vi "VXM Main Test App.vi"() -> ()   [LabVIEW 2017]
doc: "Simple Qued Message Handler type of state machine.\nAlways use this template if the VI is a UI used by a user and it is more complex than a dialog.\n(Unless you're usig something more advanced like Actor Framework)\n\nBolder Software LLC"
uses:
  Classes/UI ExecutionCtrls/UI ExecutionCtrls.lvclass
  Classes/UI MotionStatus/UI MotionStatus.lvclass
  Support/MessageAPI/MoveAllAbsolute.ctl
  Classes/UI ExecutionCtrls/MotionExecutionCtrlRefs.ctl
  Classes/UI MotionStatus/MotionStatusLEDCtrlRefs.ctl
  Classes/UI MotionStatus/PositonIndicatorsCtrlRefs.ctl
  Support/MessageQue/MessageQue.lvlib
  Support/UserEvent-ExitEventLoop/UserEvent-ExitEventLoop.lvlib
panel:
  out "Home Established":bool
  in  "Polarization":u16(ring) items=["Vertical", "Horizontal"]
  in  "Move to Pos.":bool
  in  "Position":i32=1 caption="Antenna\nPosition" min=0 max=15 step=1
  in  "clear":bool
  out "UI Messages":string
  in  "MoveAllAbsolute":bool
  out "testing 2":bool
  in  "Stop Motion":bool
  out "T moving":bool
  out "Z moving":bool
  out "Y moving":bool
  out "X moving":bool
  out "Position,steps 4":sgl caption="Angle, degrees"
  out "Position,steps 3":sgl caption="Z Position, mm"
  out "Position,steps":sgl caption="Y Position, mm"
  out "Position,steps":sgl caption="X Position, mm"
  in  "T Jog, steps":i32 caption="T Jog distance, steps"
  in  "Z Jog, steps":i32 caption="Z Jog distance, steps"
  in  "Y Jog, steps":i32 caption="Y Jog distance, steps"
  in  "X Jog, steps":i32 caption="X Jog distance, steps"
  in  "FindHomeAll":bool
  in  "HomeAll":bool
  in  "T Home Button":bool
  in  "T Jog Neg.":bool
  in  "T Jog Pos.":bool
  in  "Set T Position, Deg.":dbl format="%.4f"
  in  "Z Home Button":bool
  in  "Z Jog Neg.":bool
  in  "Z Jog Pos.":bool
  in  "Set Z Position, mm":dbl format="%.4f"
  in  "Y Home Button":bool
  in  "Y Jog Neg.":bool
  in  "Y Jog Pos.":bool
  in  "Set Y Position, mm":dbl format="%.4f"
  in  "X Home Button":bool
  in  "X Jog Neg.":bool
  in  "X Jog Pos.":bool
  in  "Set X Position, mm":dbl format="%.4f"
  in  "Generate \"DAQ\" Loop TestError":bool
  in  "test error":errorcluster
  in  "Generate \"Main\" Loop TestError":bool
  out "i event":i32=6 caption="ievent"
  out "Command":string
  out "i main":i32=6
  # "Could put jog size control\non FP here to easily \nadjust jog and implement\nrelative moves trough the\njog buttons."
  # "Could set ini file as\nmotion / no motion\nand certain controls\nwould change context"
  # "combine this with Antenna Test"
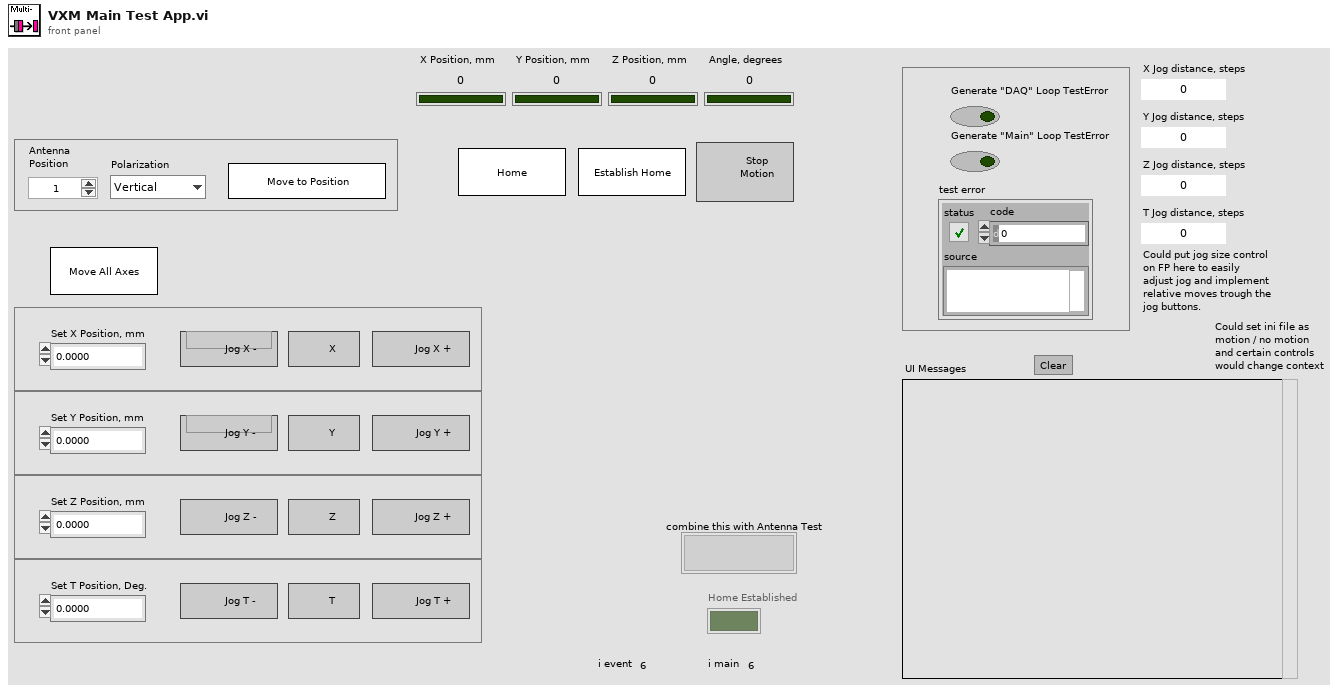
[diagram p1: front panel]
types:
  T1 = cluster{"ExecCtrls":refnum<class "UI ExecutionCtrls.lvclass">, "StatusInds":refnum<class "UI MotionStatus.lvclass">}
  T2 = typedef "MultipleMessageQues vxm.ctl" = cluster{"Main que":T3, "Error que":T3, "VXM Svc que":T3, "Listener que":T3, "VXM ACK que":T3, "DAQ que":T3}
  T3 = typedef "MessageQue.lvlib/MessageQue.ctl" = refnum<queue>
  T4 = typedef "MoveAllAbsolute.ctl" = cluster{"MoveType":string, "Move Params":dbl[]}
  T5 = typedef "PositonIndicatorsCtrlRefs.ctl" = cluster{"XPosition,steps":refnum<vi>, "YPosition,steps":refnum<vi>, "ZPosition,steps":refnum<vi>, "TPosition,steps":refnum<vi>}
  T6 = typedef "MotionStatusLEDCtrlRefs.ctl" = cluster{"Y moving":refnum<vi>, "Z moving":refnum<vi>, "T moving":refnum<vi>, "X moving":refnum<vi>}
  T7 = typedef "MotionExecutionCtrlRefs.ctl" = cluster{"MoveAllAbsolute":refnum<vi>, "Move to Pos.":refnum<vi>, "HomeAll":refnum<vi>, "FindHomeAll":refnum<vi>, "X Jog Pos.":refnum<vi>, "X Jog Neg.":refnum<vi>, "Y Jog Pos.":refnum<vi>, "Y Jog Neg. ":refnum<vi>, "Z Jog Pos.":refnum<vi>, "Z Jog Neg.":refnum<vi>, "T Jog Pos.":refnum<vi>, "T Jog Neg.":refnum<vi>, "X Home Button":refnum<vi>, "Y Home Button":refnum<vi>, "Z Home Button":refnum<vi>, "T Home Button":refnum<vi>}
  T8 = typedef "UIMessage.ctl" = cluster{"EventCode":i32, "Numeric":dbl, "String":string, "Variant":variant}
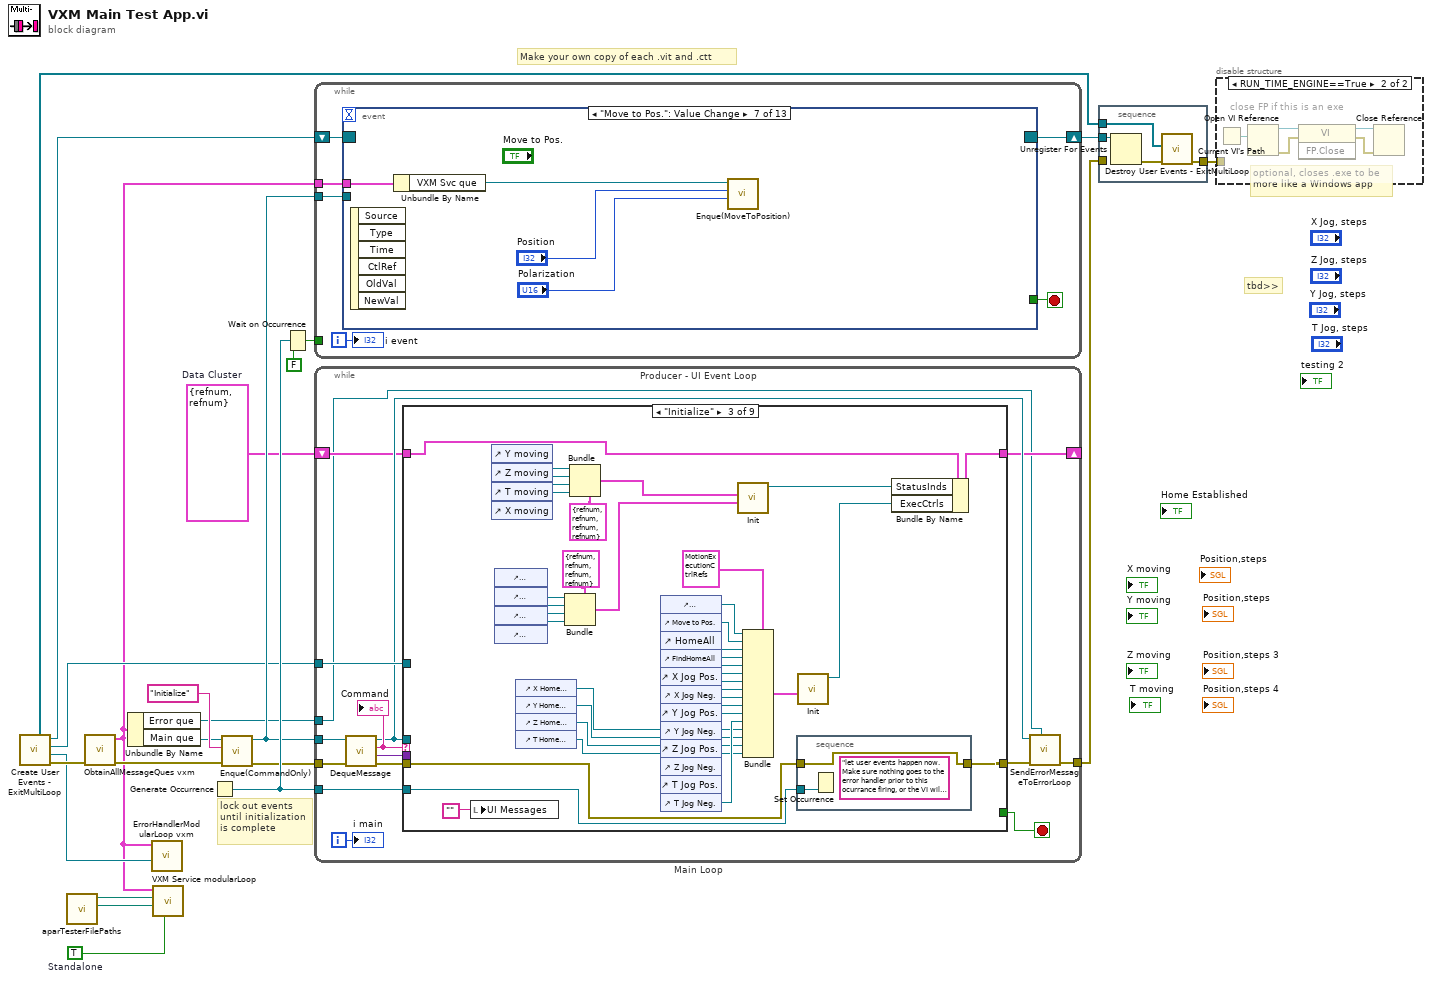
[diagram p0: block diagram]
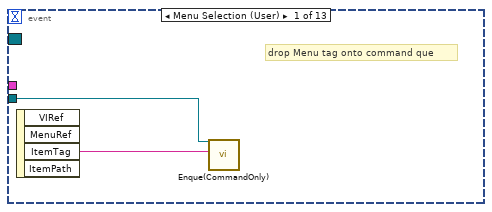
[diagram p3: hidden frame]
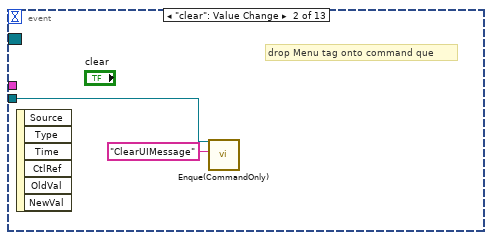
[diagram p4: hidden frame]
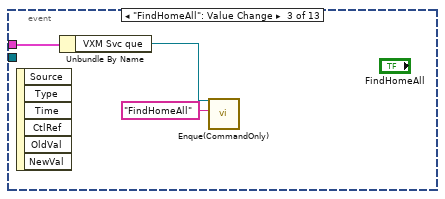
[diagram p5: hidden frame]
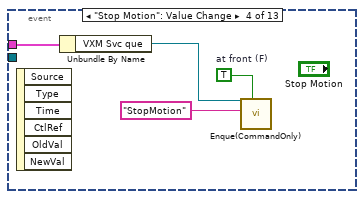
[diagram p6: hidden frame]
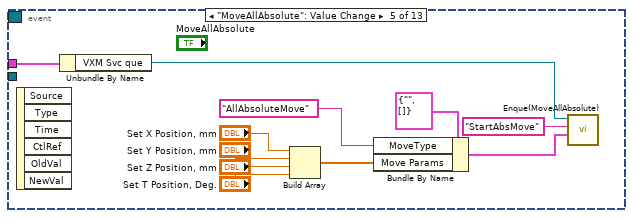
[diagram p7: hidden frame]
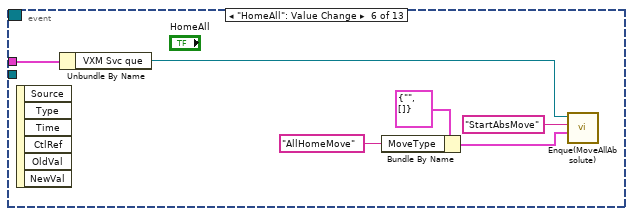
[diagram p8: hidden frame]
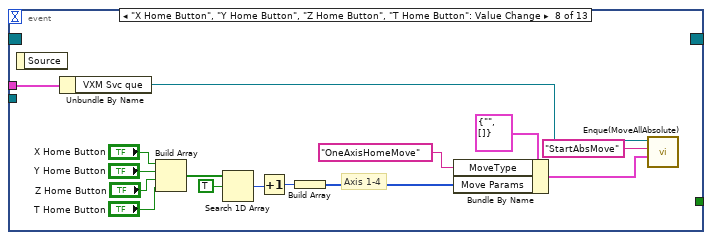
[diagram p9: hidden frame]
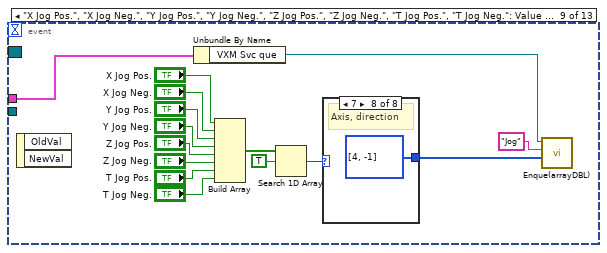
[diagram p10: hidden frame]
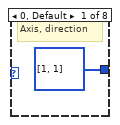
[diagram p11: hidden frame]
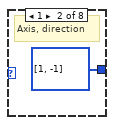
[diagram p12: hidden frame]
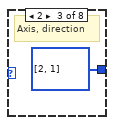
[diagram p13: hidden frame]
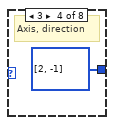
[diagram p14: hidden frame]
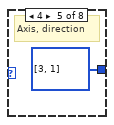
[diagram p15: hidden frame]
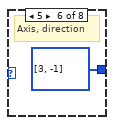
[diagram p16: hidden frame]
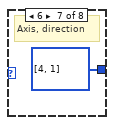
[diagram p17: hidden frame]
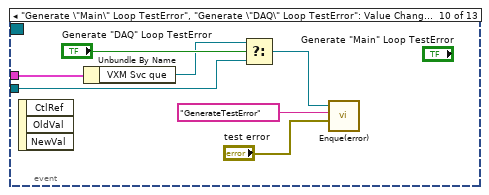
[diagram p18: hidden frame]
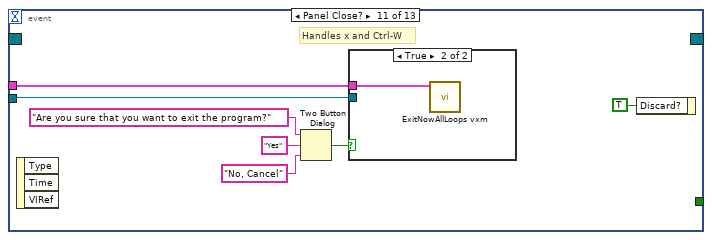
[diagram p19: hidden frame]
diagram:
  w1 = TRUE  # Standalone
  w13 = T1 {"ExecCtrls"=refnum, "StatusInds"=refnum}  # Data Cluster
  # "tbd>>"
  # "Make your own copy of each .vit and .ctt"
  # "lock out events\nuntil initialization\nis complete"
  # "optional, closes .exe to be \nmore like a Windows app"
  n1 = call "Create User Events - ExitMultiLoop.vi"() -> ("error out"=w12:errorcluster, "ExitALLLoops event out"=w5:refnum<user-event>, "ExitEventLoop event out"=w6:refnum<user-event>, "Events Registration Refnum"=w16:refnum<event-registration>, "user event array"=w7:refnum<user-event>[])  [unwired: 7 in]
  n2 = call "aparTesterFilePaths.vi"() -> ("Config File Path Motion"=w3:path, "Config File Path"=w2:path)  [unwired: 6 in, 4 out]
  n3 = call "ObtainAllMessageQues vxm.vi"("error in"=w12) -> ("error out"=w11:errorcluster, "MessageQues"=w4:T2)  [unwired: 9 in]
  n4 = Unbundle By Name(w4) -> ("Error que"=w8:T3, "Main que"=w10:T3)
  n5 = call "ErrorHandlerModularLoop vxm.vi"("exit event source"=w5, "MessageQues"=w4) -> ()  [unwired: 9 in, 1 out]
  n6 = call "VXM Service modularLoop.vi"("Standalone"=w1, "Motion Cfg File path"=w3, "Cfg File path"=w2, "MessageQues"=w4) -> ()  [unwired: 8 in]
  n7 = Generate Occurrence() -> (w22:refnum<k4>)
  n8 = call "Enque(CommandOnly).vi"("error in"=w11, "Message Command"="Initialize", "Message que"=w10) -> ("error out"=w18:errorcluster, "Message que out"=w17:T3)  [unwired: 7 in]
  n9 = Wait on Occurrence(1:FALSE ("ignore previous (T)"), 2:w22) -> (0:w15:bool)  [unwired: 1 in]
  n10 = while "Producer - UI Event Loop" {
    shift-right: [w24] -> w21
    shift-left: w16 -> [w25]
    tunnel: w17 -> [w27]
    tunnel: w15 -> [_]
    tunnel: w4 -> [w23]
    i -> [w28]
    stop <- w26 stop-if-true
    n11 = event shown="[6] \"Move to Pos.\": Value Change" {
      selector: w25 -> [_ _ _ _ _ _ _ _ _ _ _ _ _]
      dyn-events: [_ _ _ _ _ _ _ _ _ _ _ _ _] -> w24
      timeout: _ -> [_ _ _ _ _ _ _ _ _ _ _ _ _]
      tunnel: w27 -> [w29 w32 _ _ _ _ _ _ _ w100 w108 _ _]
      tunnel: [_ _ _ _ _ _ _ _ _ _ _ _ TRUE ("Discard?")] -> w26
      tunnel: w23 -> [_ _ w34 w38 w50 w56 w60 w75 w78 w103 w106 w114 _]
      event Menu Selection (User) {
        # "drop Menu tag onto command que"
        n12 = event-data() -> ("ItemTag"=w30:string)  [unwired: 1 in, 3 out]
        n13 = call "Enque(CommandOnly).vi"("Message Command"=w30, "Message que"=w29) -> ()  [unwired: 8 in, 2 out]
      }
      event "clear": Value Change {
        # "drop Menu tag onto command que"
        n14 = event-data() -> ()  [unwired: 1 in, 6 out]
        n15 = call "Enque(CommandOnly).vi"("Message Command"="ClearUIMessage", "Message que"=w32) -> ()  [unwired: 8 in, 2 out]
      }
      event "FindHomeAll": Value Change {
        n16 = event-data() -> ()  [unwired: 1 in, 6 out]
        n17 = Unbundle By Name(w34) -> ("VXM Svc que"=w35:T3)
        n18 = call "Enque(CommandOnly).vi"("Message Command"="FindHomeAll", "Message que"=w35) -> ()  [unwired: 8 in, 2 out]
      }
      event "Stop Motion": Value Change {
        w36 = TRUE  # at front (F)
        n19 = event-data() -> ()  [unwired: 1 in, 6 out]
        n20 = Unbundle By Name(w38) -> ("VXM Svc que"=w39:T3)
        n21 = call "Enque(CommandOnly).vi"("at front (F)"=w36, "Message Command"="StopMotion", "Message que"=w39) -> ()  [unwired: 7 in, 2 out]
      }
      event "MoveAllAbsolute": Value Change {
        n22 = event-data() -> ()  [unwired: 1 in, 6 out]
        n23 = Unbundle By Name(w50) -> ("VXM Svc que"=w46:T3)
        n24 = Build Array("Set X Position, mm", "Set Y Position, mm", "Set Z Position, mm", "Set T Position, Deg.") -> (w41:dbl[])
        n25 = Bundle By Name(cluster=T4 {"MoveType"="", "Move Params"=[]} ("Message Payload  array"), "MoveType"="AllAbsoluteMove", "Move Params"=w41) -> (w42:T4)
        n26 = call "Enque(MoveAllAbsolute).vi"("Message Payload  array"=w42, "Message Command"="StartAbsMove", "Message que"=w46) -> ()  [unwired: 7 in, 2 out]
      }
      event "HomeAll": Value Change {
        n27 = event-data() -> ()  [unwired: 1 in, 6 out]
        n28 = Unbundle By Name(w56) -> ("VXM Svc que"=w55:T3)
        n29 = Bundle By Name(cluster=T4 {"MoveType"="", "Move Params"=[]} ("Message Payload  array"), "MoveType"="AllHomeMove") -> (w52:T4)
        n30 = call "Enque(MoveAllAbsolute).vi"("Message Payload  array"=w52, "Message Command"="StartAbsMove", "Message que"=w55) -> ()  [unwired: 7 in, 2 out]
      }
      event "Move to Pos.": Value Change {
        n31 = event-data() -> ()  [unwired: 1 in, 6 out]
        n32 = Unbundle By Name(w60) -> ("VXM Svc que"=w59:T3)
        n33 = call "Enque(MoveToPosition).vi"("Polarization"="Polarization", "Position"="Position", "Message que"=w59) -> ()  [unwired: 7 in, 2 out]
      }
      event "X Home Button", "Y Home Button", "Z Home Button", "T Home Button": Value Change {
        # "Axis 1-4"
        n34 = event-data() -> ()  [unwired: 1 in, 1 out]
        n35 = Unbundle By Name(w75) -> ("VXM Svc que"=w74:T3)
        n36 = Build Array("X Home Button", "Y Home Button", "Z Home Button", "T Home Button") -> (w67:bool[])
        n37 = Search 1D Array(1D array=w67, element=TRUE) -> (index of element=w65:i32)  [unwired: 1 in]
        n38 = Increment(x=w65) -> (x+1=w64:i32)
        n39 = Build Array(w64) -> (w63:i32[])
        n40 = Bundle By Name(cluster=T4 {"MoveType"="", "Move Params"=[]} ("Message Payload  array"), "MoveType"="OneAxisHomeMove", "Move Params"=w63) -> (w71:T4)
        n41 = call "Enque(MoveAllAbsolute).vi"("Message Payload  array"=w71, "Message Command"="StartAbsMove", "Message que"=w74) -> ()  [unwired: 7 in, 2 out]
      }
      event "X Jog Pos.", "X Jog Neg.", "Y Jog Pos.", "Y Jog Neg.", "Z Jog Pos.", "Z Jog Neg.", "T Jog Pos.", "T Jog Neg.": Value Change {
        n42 = event-data() -> ()  [unwired: 1 in, 2 out]
        n43 = Unbundle By Name(w78) -> ("VXM Svc que"=w77:T3)
        n44 = Build Array("X Jog Pos.", "X Jog Neg.", "Y Jog Pos.", "Y Jog Neg.", "Z Jog Pos.", "Z Jog Neg.", "T Jog Pos.", "T Jog Neg.") -> (w82:bool[])
        n45 = Search 1D Array(1D array=w82, element=TRUE) -> (index of element=w80:i32)  [unwired: 1 in]
        n46 = case shown="7" w80 {
          tunnel: [i32[] [1, 1] i32[] [1, -1] i32[] [2, 1] i32[] [2, -1] i32[] [3, 1] i32[] [3, -1] i32[] [4, 1] i32[] [4, -1]] -> w79
          frame 0, Default {
            # "Axis, direction"
          }
          frame 1 {
            # "Axis, direction"
          }
          frame 2 {
            # "Axis, direction"
          }
          frame 3 {
            # "Axis, direction"
          }
          frame 4 {
            # "Axis, direction"
          }
          frame 5 {
            # "Axis, direction"
          }
          frame 6 {
            # "Axis, direction"
          }
          frame 7 {
            # "Axis, direction"
          }
        }
        n47 = call "Enque(arrayDBL).vi"("Message Payload  array"=w79, "Message Command"="Jog", "Message que"=w77) -> ()  [unwired: 7 in, 2 out]
      }
      event "Generate \"Main\" Loop TestError", "Generate \"DAQ\" Loop TestError": Value Change {
        n48 = event-data() -> ()  [unwired: 1 in, 3 out]
        n49 = Unbundle By Name(w103) -> ("VXM Svc que"=w101:T3)
        n50 = Select(t=w101, s="Generate \"DAQ\" Loop TestError", f=w100) -> (s? t:f=w99:T3)
        n51 = call "Enque(error).vi"("Message Payload  error cluster"="test error", "Message Command"="GenerateTestError", "Message que"=w99) -> ()  [unwired: 7 in, 2 out]
      }
      event Panel Close? {
        # "Handles x and Ctrl-W"
        n52 = event-data() -> ()  [unwired: 1 in, 3 out]
        n53 = Two Button Dialog(message="Are you sure that you want to exit the program?", 1:"No, Cancel" ("F button name (\"Cancel\")"), 2:"Yes" ("T button name (\"OK\")")) -> (T button?=w107:bool)
        n54 = case shown="True" w107 {
          tunnel: w108 -> [_ _]
          tunnel: w106 -> [_ w113]
          frame False {
          }
          frame True {
            n55 = call "ExitNowAllLoops vxm.vi"("MessageQues"=w113) -> ()  [unwired: 10 in, 1 out]
          }
        }
        n56 = event-data("Discard?"=TRUE) -> ()  [unwired: 1 in, 1 out]
      }
      event User Event {
        n57 = event-data() -> ()  [unwired: 1 in, 4 out]
        n58 = call "ExitNowAllLoops vxm.vi"("MessageQues"=w114) -> ()  [unwired: 10 in, 1 out]
      }
      event User Event {
        n59 = event-data() -> ()  [unwired: 1 in, 4 out]
      }
    }
    "i event" <- w28
  }
  n60 = while "Main Loop" {
    tunnel: w22 -> [w123]
    shift-right: [w118] -> _
    shift-left: w13 -> [w119]
    tunnel: w17 -> [w129]
    tunnel: w18 -> [w128]
    tunnel: w6 -> [w124]
    tunnel: [w117] -> w14
    tunnel: w8 -> [w116]
    i -> [w130]
    stop <- w122 stop-if-true
    n61 = call "DequeMessage.vi"("error in"=w128, "Message que"=w129) -> ("error out"=w126:errorcluster, "Message Payload"=w125:variant, "Message Command"=w127:string, "Message que out"=w120:T3)  [unwired: 4 in, 2 out]
    "Command" <- w127
    n62 = case shown="\"Initialize\"" w127 {
      selector: w127 -> [_ w133 _ _ _ _ _ _ _]
      tunnel: w126 -> [_ _ w152 _ _ _ _ _ w234]
      tunnel: w120 -> [_ _ _ _ _ _ _ _ w232]
      tunnel: w125 -> [_ _ _ w185 _ w224 w227 _ _]
      tunnel: w124 -> [_ _ _ _ _ _ _ _ w230]
      tunnel: w123 -> [_ _ w153 _ _ _ _ _ _]
      tunnel: [_ _ w174 _ _ _ w226 _ _] -> w121
      tunnel: [_ _ _ _ _ _ _ _ TRUE] -> w122
      tunnel: [w131 w132 w143 w179 w220 w225 w228 w229 w231] -> w118
      tunnel: w119 -> [w131 w132 w151 w180 w220 w225 w228 w229 w231]
      frame "idle" {
      }
      frame Default {
        # "handles erroneous command strings"
        n63 = Concatenate Strings("WARNING\n" ("message"), w133, " is not a case in this VI" ("message")) -> (w136:string)
        n64 = One Button Dialog(message=w136) -> ()  [unwired: 1 in, 1 out]
      }
      frame "Initialize" {
        n65 = local write "UI Messages"("") -> ()
        n66 = control-ref of="Y moving"() -> (w172:refnum<vi>)
        n67 = control-ref of="Z moving"() -> (w171:refnum<vi>)
        n68 = control-ref of="T moving"() -> (w170:refnum<vi>)
        n69 = control-ref of="X moving"() -> (w169:refnum<vi>)
        n70 = control-ref of="Position,steps"() -> (w168:refnum<vi>)
        n71 = control-ref of="Position,steps"() -> (w167:refnum<vi>)
        n72 = control-ref of="Position,steps 3"() -> (w166:refnum<vi>)
        n73 = control-ref of="Position,steps 4"() -> (w165:refnum<vi>)
        n74 = control-ref of="X Home Button"() -> (w140:refnum<vi>)
        n75 = control-ref of="Y Home Button"() -> (w139:refnum<vi>)
        n76 = control-ref of="Z Home Button"() -> (w138:refnum<vi>)
        n77 = control-ref of="T Home Button"() -> (w137:refnum<vi>)
        n78 = Bundle(cluster=T5 {"XPosition,steps"=refnum, "YPosition,steps"=refnum, "ZPosition,steps"=refnum, "TPosition,steps"=refnum} ("PositionIndCtrls"), "XPosition,steps"=w168, "YPosition,steps"=w167, "ZPosition,steps"=w166, "TPosition,steps"=w165) -> (w144:T5)
        n79 = Bundle(cluster=T6 {"Y moving"=refnum, "Z moving"=refnum, "T moving"=refnum, "X moving"=refnum} ("MotionStatusCtrls"), "Y moving"=w172, "Z moving"=w171, "T moving"=w170, "X moving"=w169) -> (w147:T6)
        n80 = control-ref of="MoveAllAbsolute"() -> (w150:refnum<vi>)
        n81 = control-ref of="Move to Pos."() -> (w154:refnum<vi>)
        n82 = control-ref of="HomeAll"() -> (w155:refnum<vi>)
        n83 = control-ref of="FindHomeAll"() -> (w156:refnum<vi>)
        n84 = control-ref of="X Jog Pos."() -> (w157:refnum<vi>)
        n85 = control-ref of="X Jog Neg."() -> (w158:refnum<vi>)
        n86 = control-ref of="Y Jog Pos."() -> (w159:refnum<vi>)
        n87 = control-ref of="Y Jog Neg."() -> (w160:refnum<vi>)
        n88 = control-ref of="Z Jog Pos."() -> (w161:refnum<vi>)
        n89 = control-ref of="Z Jog Neg."() -> (w162:refnum<vi>)
        n90 = control-ref of="T Jog Pos."() -> (w163:refnum<vi>)
        n91 = control-ref of="T Jog Neg."() -> (w164:refnum<vi>)
        n92 = call "Init.vi"("PositionIndCtrls"=w144, "MotionStatusCtrls"=w147) -> ("UI MotionStatus out"=w142:refnum<class "UI MotionStatus.lvclass">)  [unwired: 8 in, 1 out]
        n93 = Bundle(cluster=T7 {"MoveAllAbsolute"=refnum, "Move to Pos."=refnum, "HomeAll"=refnum, "FindHomeAll"=refnum, "X Jog Pos."=refnum, "X Jog Neg."=refnum, "Y Jog Pos."=refnum, "Y Jog Neg. "=refnum, "Z Jog Pos."=refnum, "Z Jog Neg."=refnum, "T Jog Pos."=refnum, "T Jog Neg."=refnum, "X Home Button"=refnum, "Y Home Button"=refnum, "Z Home Button"=refnum, "T Home Button"=refnum} ("ExecCtrlRefs"), "MoveAllAbsolute"=w150, "Move to Pos."=w154, "HomeAll"=w155, "FindHomeAll"=w156, "X Jog Pos."=w157, "X Jog Neg."=w158, "Y Jog Pos."=w159, "Y Jog Neg."=w160, "Z Jog Pos."=w161, "Z Jog Neg."=w162, "T Jog Pos."=w163, "T Jog Neg."=w164, "X Home Button"=w140, "Y Home Button"=w139, "Z Home Button"=w138, "T Home Button"=w137) -> (w148:T7)
        n94 = stacked-sequence {
          tunnel: w152 -> [w175]
          tunnel: [w175] -> w174
          tunnel: w153 -> [w176]
          frame #0 {
            (unwired) "let user events happen now. Make sure nothing goes to the error handler prior to this ocurrance firing, or the VI will be frozen."
            n95 = Set Occurrence(w176) -> ()
          }
        }
        n96 = call "Init.vi"("ExecCtrlRefs"=w148) -> ("UI ExecutionCtrls out"=w141:refnum<class "UI ExecutionCtrls.lvclass">)  [unwired: 9 in, 1 out]
        n97 = Bundle By Name(cluster=w151, "StatusInds"=w142, "ExecCtrls"=w141) -> (w143:T1)
      }
      frame "UIMessage" {
        # "for debug"
        n98 = call "ConvertTo(UIMessage).vi"("Message Payload"=w185) -> ("UIMsg"=w182:T8)  [unwired: 9 in, 1 out]
        n99 = local read "UI Messages"() -> (w184:string)
        n100 = Unbundle By Name(w182) -> ("EventCode"=w181:i32, "Numeric"=w178:dbl, "String"=w177:string)  [unwired: 1 out]
        n101 = case shown="104" w181 {
          tunnel: w180 -> [w186 w190 w194 w200 w208 w217]
          tunnel: [w186 w190 w194 w200 w208 w217] -> w179
          tunnel: w178 -> [_ w187 w191 _ _ _]
          tunnel: w177 -> [_ _ _ w199 w207 w216]
          frame -1, Default {
          }
          frame 100 {
            # "100 Motion Started"
            n102 = Unbundle By Name(w190) -> ("ExecCtrls"=w188:refnum<class "UI ExecutionCtrls.lvclass">, "StatusInds"=w189:refnum<class "UI MotionStatus.lvclass">)
            n103 = call "StartMotion.vi"("Axis, 1 - 4"=w187, "UI MotionStatus in"=w189) -> ()  [unwired: 8 in, 2 out]
            n104 = call "StartMotion.vi"("UI ExecutionCtrls in"=w188) -> ()  [unwired: 9 in, 2 out]
          }
          frame 101 {
            # "101 Motion Stopped"
            n105 = Unbundle By Name(w194) -> ("ExecCtrls"=w192:refnum<class "UI ExecutionCtrls.lvclass">, "StatusInds"=w193:refnum<class "UI MotionStatus.lvclass">)
            n106 = call "StopMotion.vi"("Axis, 1 - 4"=w191, "UI MotionStatus in"=w193) -> ()  [unwired: 8 in, 2 out]
            n107 = call "StopMotion.vi"("UI ExecutionCtrls in"=w192) -> ()  [unwired: 9 in, 2 out]
          }
          frame 102 {
            # "102 Stop Motion command invoked"
            n108 = Unbundle By Name(w200) -> ("ExecCtrls"=w201:refnum<class "UI ExecutionCtrls.lvclass">, "StatusInds"=w202:refnum<class "UI MotionStatus.lvclass">)
            n109 = Spreadsheet String To Array(delimiter (Tab)=",", format string="%.5f", spreadsheet string=w199, array type (2D Dbl)=dbl[] []) -> (array=w195:dbl[])
            n110 = call "WriteAllPositions.vi"("Positions, counts"=w195, "UI MotionStatus in"=w202) -> ()  [unwired: 8 in, 2 out]
            n111 = call "StopMotion.vi"("UI ExecutionCtrls in"=w201) -> ()  [unwired: 9 in, 2 out]
          }
          frame 103 {
            # "update all four positions, position only not LEDs"
            n112 = Unbundle By Name(w208) -> ("StatusInds"=w209:refnum<class "UI MotionStatus.lvclass">)
            n113 = Spreadsheet String To Array(delimiter (Tab)=",", format string="%.5f", spreadsheet string=w207, array type (2D Dbl)=dbl[] []) -> (array=w203:dbl[])
            n114 = call "WriteAllPositions.vi"("Positions, counts"=w203, "UI MotionStatus in"=w209) -> ()  [unwired: 8 in, 2 out]
          }
          frame 104 {
            # "104 update one position"
            n115 = Unbundle By Name(w217) -> ("StatusInds"=w218:refnum<class "UI MotionStatus.lvclass">)
            n116 = Spreadsheet String To Array(delimiter (Tab)=",", format string="%.5f", spreadsheet string=w216, array type (2D Dbl)=dbl[] []) -> (array=w212:dbl[])
            n117 = Index Array(array=w212) -> (element #1=w210:dbl, element #2=w211:dbl)  [unwired: 2 in]
            n118 = call "WriteOnePosition.vi"("Axis, 1 - 4"=w210, "Position, counts"=w211, "UI MotionStatus in"=w218) -> ()  [unwired: 7 in, 2 out]
          }
        }
        n119 = call "ListenerForMotion.vi"("UIMsg"=w182, "UI Messages"=w184) -> ("String"=→"UI Messages":string)  [unwired: 9 in]
      }
      frame "ClearUIMessage" {
        n120 = local write "UI Messages"("") -> ()
      }
      frame "ClearError" {
        n121 = call "ConvertTo(error).vi"("Message Payload"=w224) -> ("Message Payload error"=w223:errorcluster)  [unwired: 9 in, 1 out]
        n122 = Unbundle By Name(w223) -> ("code"=w222:i32, "source"=w221:string)
        n123 = case shown="1" w222 {
          tunnel: w221 -> [_ _]
          frame 0, Default {
          }
          frame 1 {
            # "could take error action here\nfor selected error codes, and\nignore all other codes"
          }
        }
      }
      frame "GenerateTestError" {
        n124 = call "ConvertTo(error).vi"("Message Payload"=w227) -> ("Message Payload error"=w226:errorcluster)  [unwired: 9 in, 1 out]
      }
      frame "---Copy This Frame---" {
        # "Duplicate this frame when creating new messages.  Change this comment in the duplicated frame to describe this message."
      }
      frame "ExitNow" {
        # "Release the message \nque reference"
        n125 = call "Fire User Event - ExitEventLoop.vi"("user event ExitEventLoop"=w230) -> ()  [unwired: 10 in, 1 out]
        n126 = Release Queue(queue=w232, error in (no error)=w234) -> ()  [unwired: 1 in, 3 out]
      }
    }
    n127 = call "SendErrorMessageToErrorLoop.vi"("Error Message que"=w116, "error in (no error)"=w121, "Loop Message que"=w120) -> ("error out"=w117:errorcluster)  [unwired: 8 in]
    "i main" <- w130
  }
  n128 = stacked-sequence {
    tunnel: w21 -> [w238]
    tunnel: [w236] -> w20
    tunnel: w7 -> [w235]
    tunnel: w14 -> [_]
    frame #0 {
      n129 = Unregister For Events(event registration refnum=w238) -> (error out=w237:errorcluster)  [unwired: 1 in]
      n130 = call "Destroy User Events - ExitMultiLoop.vi"("error in (no error)"=w237, "user event array"=w235) -> ("error out"=w236:errorcluster)  [unwired: 9 in]
    }
  }
  n131 = disable-structure "Conditional Disable Structure" shown="RUN_TIME_ENGINE==True" {
    disable-tunnel: w20 -> [_ _]
    frame condition #0 (active) {
    }
    frame condition #1 {
      # "close FP if this is an exe"
      n132 = Current VI's Path() -> (path=w243:path)
      n133 = Open VI Reference(vi path=w243) -> (vi reference=w239:refnum<vi>, error out=w242:errorcluster)  [unwired: 5 in]
      n134 = invoke on="Invoke Node" class="VI" method="FP.Close"(reference=w239, error in=w242) -> (reference out=w240:refnum<vi>, error out=w241:errorcluster)  [unwired: 1 in, 1 out]
      n135 = Close Reference(reference=w240, error in (no error)=w241) -> ()  [unwired: 1 out]
    }
  }
